vi "Open Weekly Save File.vi"(8 "error in (no error)":errorcluster, 11 "Data recording root path":path) -> (0 "error out":errorcluster, 3 "Daily datafile":T1 format="%.0x")   [LabVIEW 2016]
uses:
  <vilib>/addons/h5labview2/base/hid_t.ctl
  <vilib>/addons/h5labview2/file/H5Fmode.ctl
  <vilib>/addons/h5labview2/file/H5F.lvlib
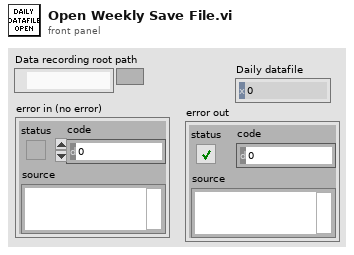
[diagram p1: front panel]
types:
  T1 = typedef "hid_t.ctl" = i32
  T2 = typedef "H5F.lvlib/H5Fmode.ctl" = enum16{"read-only", "read-write", "overwrite", "create new", "open or create"}
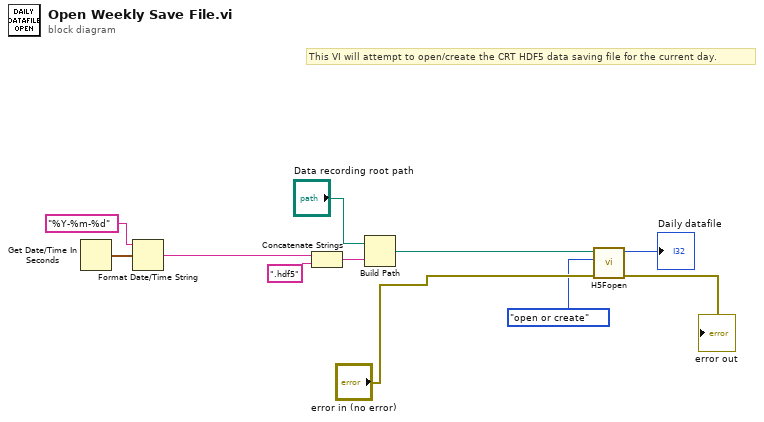
[diagram p0: block diagram]
diagram:
  # "This VI will attempt to open/create the CRT HDF5 data saving file for the current day."
  n1 = Get Date/Time In Seconds() -> (seconds since 1Jan1904=w2:timestamp)
  n2 = Format Date/Time String(time format string (%c)="%Y-%m-%d", seconds (now)=w2) -> (date/time string=w11:string)  [unwired: 1 in]
  n3 = Concatenate Strings(w11, ".hdf5" ("string")) -> (w9:string)
  n4 = Build Path(base path="Data recording root path", name or relative path=w9) -> (appended path=w5:path)
  n5 = call <vilib>:"H5Fopen.vi"("error in (no error)"="error in (no error)", "mode (read-only)"=H5Fmode."open or create", "path"=w5) -> ("error out"=→"error out":errorcluster, "ref out"=→"Daily datafile":T1)  [unwired: 7 in]
